vi "set scanning speed.vi"(8 "error in (no error)":errorcluster, 11 "DAQOrcaFlash in":refnum<class "DAQOrcaFlash.lvclass">) -> (0 "error out":errorcluster, 3 "DAQOrcaFlash out":refnum<class "DAQOrcaFlash.lvclass">)   [LabVIEW 2012, in "DAQOrcaFlash.lvclass"]
uses:
  DAQOrcaFlash.lvclass
  DAQOrcaFlash.lvclass/DAQOrcaFlash.ctl
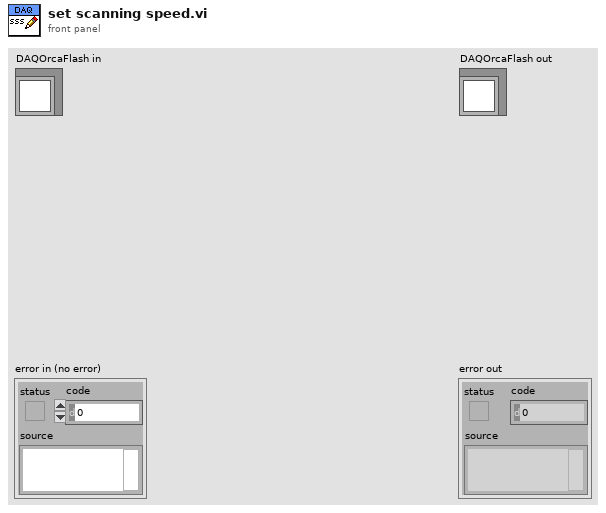
[diagram p1: front panel]
types:
  T1 = typedef "DAQOrcaFlash.lvclass/sensor_mode.ctl" = sgl
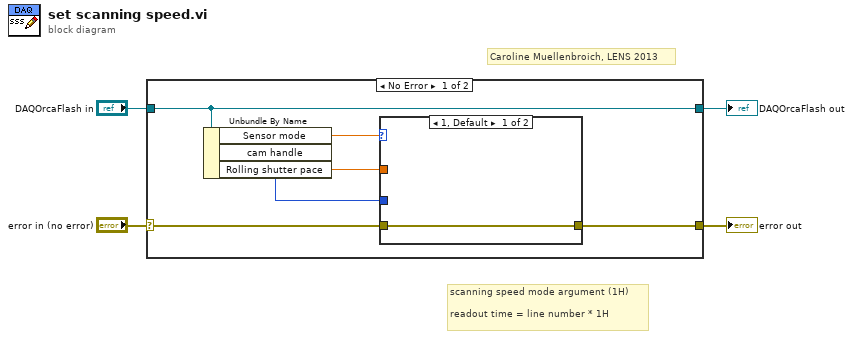
[diagram p0: block diagram]
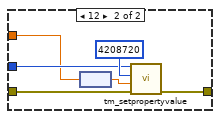
[diagram p2: hidden frame]
diagram:
  # "scanning speed mode argument (1H)\n\nreadout time = line number * 1H"
  # "Caroline Muellenbroich, LENS 2013"
  n1 = case shown="No Error" "error in (no error)" {
    selector: "error in (no error)" -> [w8 w19]
    tunnel: [w9 w19] -> w3
    tunnel: [w10 w18] -> w1
    tunnel: "DAQOrcaFlash in" -> [w10 w18]
    frame No Error {
      n2 = Unbundle By Name(w10) -> ("Sensor mode"=w5:T1, "cam handle"=w7:u32, "Rolling shutter pace"=w6:sgl[unit])
      n3 = case shown="1, Default" w5 {
        tunnel: [w11 w17] -> w9
        tunnel: w8 -> [w11 w15]
        tunnel: w7 -> [_ w14]
        tunnel: w6 -> [_ w13]
        frame 1, Default {
        }
        frame 12 {
          n4 = node(w13) -> (w12:sgl)
          n5 = call <userlib>:"tm_setpropertyvalue.vi"("error in (no error)"=w15, "Value in"=w12, "Property ID"=u32 4208720, "Handle in"=w14) -> ("error out"=w17:errorcluster)  [unwired: 6 in, 1 out]
        }
      }
    }
    frame Error {
    }
  }
  "error out" <- w3
  "DAQOrcaFlash out" <- w1
